vi "Count Up.vi"(8 "error in":errorcluster, 9 "preset value":u32=10, 10 "reset":bool, 11 "count up":bool) -> (0 "error out":errorcluster, 2 "counter value":u32, 3 "done":bool)   [LabVIEW 2020, in "NI_FunctionBlock Libraries.lvlib"]
uses:
  <vilib>/functionblocks/NI_FunctionBlock Libraries.lvlib
  <vilib>/ptbypt/NI_PtbyPt.lvlib
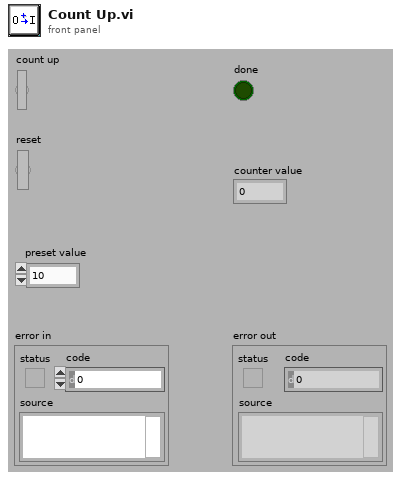
[diagram p1: front panel]
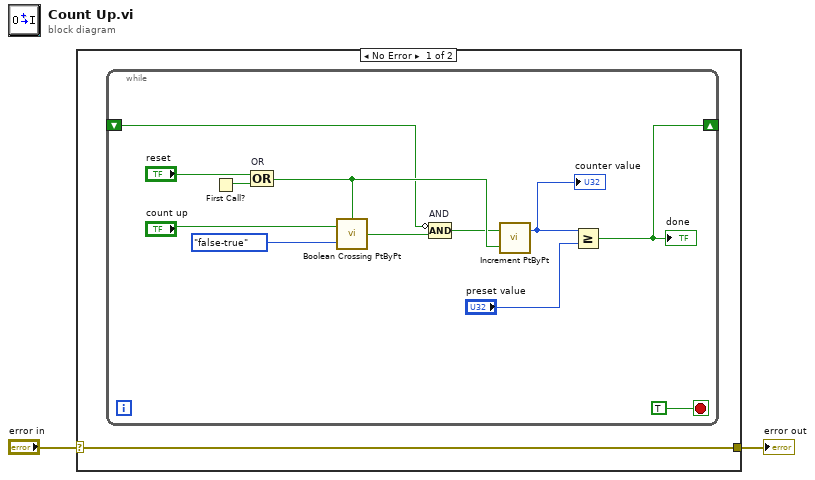
[diagram p0: block diagram]
diagram:
  n1 = case shown="No Error" "error in" {
    selector: "error in" -> [w3 w16]
    tunnel: [w3 w16] -> w1
    frame No Error {
      n2 = while {
        shift-right: [w6] -> _
        shift-left: _ -> [w5]
        stop <- TRUE stop-if-true
        n3 = First Call?() -> (First Call?: T/F=w12:bool)
        n4 = Compound Arithmetic op=OR "OR"("reset", w12) -> (w11:bool)
        n5 = call <vilib>:"Boolean Crossing PtByPt.vi"("initialize"=w11, "direction"=enum16{"either", "false-true", "true-false"}."false-true", "input"="count up") -> ("crossing"=w4:bool)
        n6 = Compound Arithmetic op=AND "AND"(invert w5, w4) -> (w7:bool)
        n7 = call <vilib>:"Increment PtByPt.vi"("initialize"=w11, "activate"=w7) -> ("counter"=w9:u32)  [unwired: 1 out]
        "counter value" <- w9
        n8 = Greater Or Equal?(x=w9, y="preset value") -> (x >= y?=w6:bool)
        "done" <- w6
      }
    }
    frame Error {
    }
  }
  "error out" <- w1
